vi "Teardown.vi"(7 "Queue Actor in":refnum<class "Queue Actor.lvclass">, 11 "Error State in":refnum<class "Error State.lvclass">) -> (5 "Queue Actor out":refnum<class "Queue Actor.lvclass">)   [LabVIEW 2021, in "jettl.lvlib" / "jettl Queue Actor.lvlib" / "Error State.lvclass"]
uses:
  Error State.lvclass
  Actor/Queue Actor/Queue Actor.lvclass
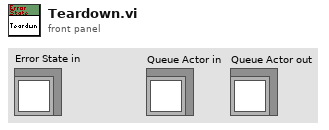
[diagram p1: front panel]
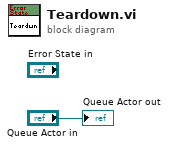
[diagram p0: block diagram]
diagram:
  "Queue Actor out" <- "Queue Actor in"
